vi "Master Sensor Update.vi"(11 "Input":T1={"GyroDevRef"={"DevStatus"={"status"=FALSE, "code"=0, "source"=""}, "Analog Channel"=enum."AI 1", "Offset"=0.0, "Gain (VoltsPerDegree/Second)"=0.0, "Gyro Type"=enum."Analog", "Handle"=0, "SPI Bus"=enum."Invalid", "Device Found"=FALSE, "Sample Rate"=1.0, "Calibrate On Open"=FALSE}, "Left Arm Limit DigitalInputDevRef"={"DevStatus"={"status"=FALSE, "code"=0, "source"=""}, "DIO Channel"=enum."DIO 1"}, "Right Arm Limit DigitalInputDevRef"={"DevStatus"={"status"=FALSE, "code"=0, "source"=""}, "DIO Channel"=enum."DIO 1"}, "Left Arm EncoderDevRef"={"DevStatus"={"status"=FALSE, "code"=0, "source"=""}, "EncoderIndex"=enum."Invalid", "CounterIndex"=enum."Invalid", "DistancePerCount"=1.0, "Decoding Type"=enum."4x"}, "Right Arm EncoderDevRef"={"DevStatus"={"status"=FALSE, "code"=0, "source"=""}, "EncoderIndex"=enum."Invalid", "CounterIndex"=enum."Invalid", "DistancePerCount"=1.0, "Decoding Type"=enum."4x"}, "Left Drive EncoderDevRef"={"DevStatus"={"status"=FALSE, "code"=0, "source"=""}, "EncoderIndex"=enum."Invalid", "CounterIndex"=enum."Invalid", "DistancePerCount"=1.0, "Decoding Type"=enum."4x"}, "Right Drive EncoderDevRef"={"DevStatus"={"status"=FALSE, "code"=0, "source"=""}, "EncoderIndex"=enum."Invalid", "CounterIndex"=enum."Invalid", "DistancePerCount"=1.0, "Decoding Type"=enum."4x"}, "BoB Photoeye DigitalInputDevRef"={"DevStatus"={"status"=FALSE, "code"=0, "source"=""}, "DIO Channel"=enum."DIO 1"}, "Range SonarMB1010AnalogDevRef"={"AIDeviceRef"={"DevStatus"={"status"=FALSE, "code"=0, "source"=""}, "Analog Channel"=enum."Invalid"}, "Scaling factor (V/in)"=0.0098, "Average Bits"=3}, "Shooter CounterDevRef"={"DevStatus"={"status"=FALSE, "code"=0, "source"=""}, "CntIndex"=enum."Invalid"}, "AccelerometerDevRef"={"DevStatus"={"status"=FALSE, "code"=0, "source"=""}, "Scaling"={"Gain (VoltsPerG)"=0.0, "Center Voltage"=0.0}, "Analog Channels"={"X-Axis"=enum."Invalid", "Y-Axis"=enum."Invalid", "Z-Axis"=enum."Invalid"}, "I2C Bus"=enum."Invalid", "SPI Bus"=enum."Invalid", "Accel Range"=0, "ADXL Axes"={"X-Axis"=FALSE, "Y-Axis"=FALSE, "Z-Axis"=FALSE}, "Handle"=0, "Device Address"=0, "Accel Type"=enum."Analog"}, "Left Hanging Erecter EncoderDevRef"={"DevStatus"={"status"=FALSE, "code"=0, "source"=""}, "EncoderIndex"=enum."Enc 0", "CounterIndex"=enum."Invalid", "DistancePerCount"=1.0, "Decoding Type"=enum."4x"}, "Right Hanging Erecter EncoderDevRef"={"DevStatus"={"status"=FALSE, "code"=0, "source"=""}, "EncoderIndex"=enum."Enc 1", "CounterIndex"=enum."Invalid", "DistancePerCount"=1.0, "Decoding Type"=enum."4x"}, "TestDigitalInputDevRef"={"DevStatus"={"status"=FALSE, "code"=0, "source"=""}, "DIO Channel"=enum."DIO 1"}} {"AccelerometerDevRef"."Device Address" format="%.0x"; "AccelerometerDevRef"."Accel Range" items=["+/- 2 g", "+/- 4 g", "+/- 8 g", "+/- 16 g"]; "Range SonarMB1010AnalogDevRef"."Average Bits" max=15; "GyroDevRef"."Sample Rate" min=0.25 max=100.0 step=0.25}) -> (3 "Output":T1={"GyroDevRef"={"DevStatus"={"status"=FALSE, "code"=0, "source"=""}, "Analog Channel"=enum."AI 1", "Offset"=0.0, "Gain (VoltsPerDegree/Second)"=0.0, "Gyro Type"=enum."Analog", "Handle"=0, "SPI Bus"=enum."Invalid", "Device Found"=FALSE, "Sample Rate"=1.0, "Calibrate On Open"=FALSE}, "Left Arm Limit DigitalInputDevRef"={"DevStatus"={"status"=FALSE, "code"=0, "source"=""}, "DIO Channel"=enum."DIO 1"}, "Right Arm Limit DigitalInputDevRef"={"DevStatus"={"status"=FALSE, "code"=0, "source"=""}, "DIO Channel"=enum."DIO 1"}, "Left Arm EncoderDevRef"={"DevStatus"={"status"=FALSE, "code"=0, "source"=""}, "EncoderIndex"=enum."Invalid", "CounterIndex"=enum."Invalid", "DistancePerCount"=1.0, "Decoding Type"=enum."4x"}, "Right Arm EncoderDevRef"={"DevStatus"={"status"=FALSE, "code"=0, "source"=""}, "EncoderIndex"=enum."Invalid", "CounterIndex"=enum."Invalid", "DistancePerCount"=1.0, "Decoding Type"=enum."4x"}, "Left Drive EncoderDevRef"={"DevStatus"={"status"=FALSE, "code"=0, "source"=""}, "EncoderIndex"=enum."Invalid", "CounterIndex"=enum."Invalid", "DistancePerCount"=1.0, "Decoding Type"=enum."4x"}, "Right Drive EncoderDevRef"={"DevStatus"={"status"=FALSE, "code"=0, "source"=""}, "EncoderIndex"=enum."Invalid", "CounterIndex"=enum."Invalid", "DistancePerCount"=1.0, "Decoding Type"=enum."4x"}, "BoB Photoeye DigitalInputDevRef"={"DevStatus"={"status"=FALSE, "code"=0, "source"=""}, "DIO Channel"=enum."DIO 1"}, "Range SonarMB1010AnalogDevRef"={"AIDeviceRef"={"DevStatus"={"status"=FALSE, "code"=0, "source"=""}, "Analog Channel"=enum."Invalid"}, "Scaling factor (V/in)"=0.0098, "Average Bits"=3}, "Shooter CounterDevRef"={"DevStatus"={"status"=FALSE, "code"=0, "source"=""}, "CntIndex"=enum."Invalid"}, "AccelerometerDevRef"={"DevStatus"={"status"=FALSE, "code"=0, "source"=""}, "Scaling"={"Gain (VoltsPerG)"=0.0, "Center Voltage"=0.0}, "Analog Channels"={"X-Axis"=enum."Invalid", "Y-Axis"=enum."Invalid", "Z-Axis"=enum."Invalid"}, "I2C Bus"=enum."Invalid", "SPI Bus"=enum."Invalid", "Accel Range"=0, "ADXL Axes"={"X-Axis"=FALSE, "Y-Axis"=FALSE, "Z-Axis"=FALSE}, "Handle"=0, "Device Address"=0, "Accel Type"=enum."Analog"}, "Left Hanging Erecter EncoderDevRef"={"DevStatus"={"status"=FALSE, "code"=0, "source"=""}, "EncoderIndex"=enum."Enc 0", "CounterIndex"=enum."Invalid", "DistancePerCount"=1.0, "Decoding Type"=enum."4x"}, "Right Hanging Erecter EncoderDevRef"={"DevStatus"={"status"=FALSE, "code"=0, "source"=""}, "EncoderIndex"=enum."Enc 1", "CounterIndex"=enum."Invalid", "DistancePerCount"=1.0, "Decoding Type"=enum."4x"}, "TestDigitalInputDevRef"={"DevStatus"={"status"=FALSE, "code"=0, "source"=""}, "DIO Channel"=enum."DIO 1"}} {"AccelerometerDevRef"."Device Address" format="%.0x"; "AccelerometerDevRef"."Accel Range" items=["+/- 2 g", "+/- 4 g", "+/- 8 g", "+/- 16 g"]; "Range SonarMB1010AnalogDevRef"."Average Bits" max=15; "GyroDevRef"."Sample Rate" min=0.25 max=100.0 step=0.25})   [LabVIEW 2015]
uses:
  Sensors.ctl
  <vilib>/Rock Robotics/WPI/Gyro/WPI_GyroDevRef.ctl
  <vilib>/Rock Robotics/SystemInterfaces/AI/FPGA_AIChannel.ctl
  <vilib>/Rock Robotics/SystemInterfaces/spilib/spi_bus.ctl
  <vilib>/Rock Robotics/WPI/DigitalInput/WPI_DigitalInputDevRef.ctl
  <vilib>/Rock Robotics/SystemInterfaces/DIO/FPGA_DIOChannel.ctl
  <vilib>/Rock Robotics/WPI/Encoder/WPI_EncoderDevRef.ctl
  <vilib>/Rock Robotics/SystemInterfaces/Encoder/FPGA_EncoderIdx.ctl
  <vilib>/Rock Robotics/SystemInterfaces/Counter/FPGA_CounterCtrSystemIndex.ctl
  <vilib>/Rock Robotics/WPI/Encoder/WPI_EncoderType.ctl
  <vilib>/Rock Robotics/WPI/Ultrasonic/WPI_SonarMB1010AnalogDeviceRef.ctl
  <vilib>/Rock Robotics/WPI/AnalogChannel/WPI_AnalogChannelDevRef.ctl
  <vilib>/Rock Robotics/WPI/Counter/WPI_CounterDevRef.ctl
  <vilib>/Rock Robotics/WPI/Accelerometer/WPI_AccelerometerDevRef.ctl
  <vilib>/Rock Robotics/WPI/Accelerometer/WPI_AccelerometerScaling.ctl
  <vilib>/Rock Robotics/WPI/Accelerometer/WPI_AccelerometerAnalogChannels.ctl
  <vilib>/Rock Robotics/SystemInterfaces/i2clib/i2c_bus.ctl
  <vilib>/Rock Robotics/WPI/Accelerometer/ADXL345 Range.ctl
  <vilib>/Rock Robotics/WPI/Accelerometer/WPI_AccelerometerADXL345 Axes.ctl
  <vilib>/Rock Robotics/Network Tables/NT Write Number.vi
  <vilib>/Rock Robotics/Network Tables/NT Read Numeric Array.vi
  <vilib>/Rock Robotics/Network Tables/NT Write Boolean.vi
  <vilib>/Rock Robotics/Network Tables/NT Read Boolean.vi
  Robot Values.vi
  <vilib>/Rock Robotics/WPI/Ultrasonic/WPI_SonarMB1010AnalogGetRange.vi
panel:
  in  "Gyro Multiplier":dbl=1.125 format="%#_13g"
  # "ADXL"
  # "Analog"
  # "Analog"
  # "XRS"
  # "ADXL"
  # "Analog"
  # "Analog"
  # "XRS"
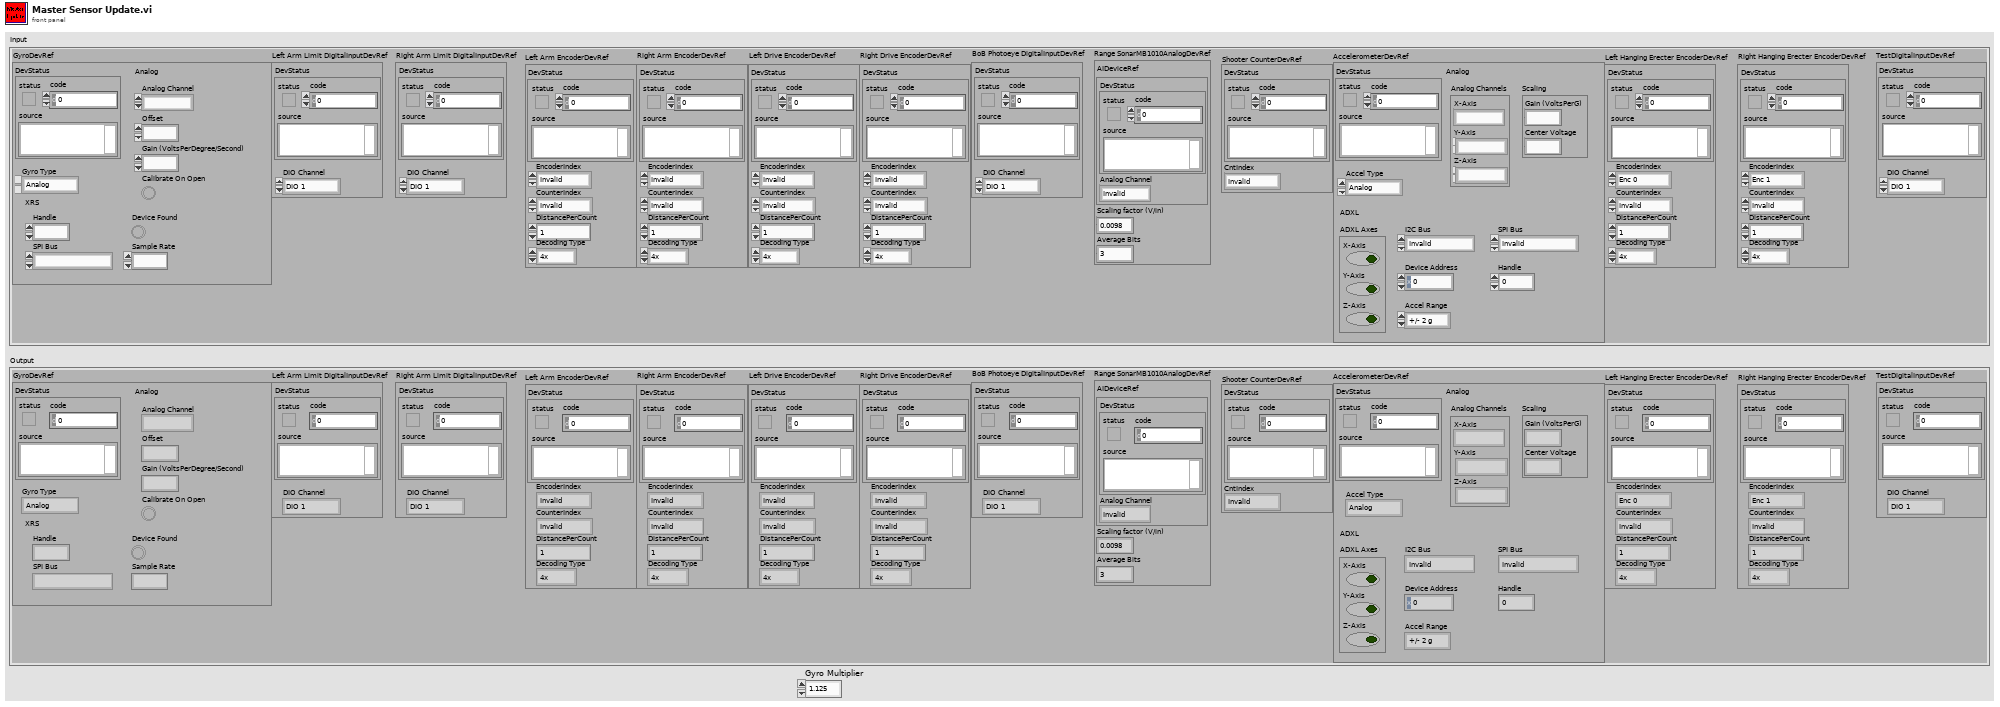
[diagram p1: front panel]
types:
  T1 = typedef "Sensors.ctl" = cluster{"GyroDevRef":T2, "Left Arm Limit DigitalInputDevRef":T5, "Right Arm Limit DigitalInputDevRef":T5, "Left Arm EncoderDevRef":T7, "Right Arm EncoderDevRef":T7, "Left Drive EncoderDevRef":T7, "Right Drive EncoderDevRef":T7, "BoB Photoeye DigitalInputDevRef":T5, "Range SonarMB1010AnalogDevRef":T11, "Shooter CounterDevRef":T13, "AccelerometerDevRef":T14, "Left Hanging Erecter EncoderDevRef":T7, "Right Hanging Erecter EncoderDevRef":T7, "TestDigitalInputDevRef":T5}
  T2 = typedef "WPI_GyroDevRef.ctl" = cluster{"DevStatus":errorcluster, "Analog Channel":T3, "Offset":dbl, "Gain (VoltsPerDegree/Second)":dbl, "Gyro Type":enum16{"Analog", "XRS450"}, "Handle":i32, "SPI Bus":T4, "Device Found":bool, "Sample Rate":dbl, "Calibrate On Open":bool}
  T3 = typedef "FPGA_AIChannel.ctl" = enum8{"AI 0", "AI 1", "AI 2", "AI 3", "AI MXP 0", "AI MXP 1", "AI MXP 2", "AI MXP 3", "Invalid"}
  T4 = typedef "spi_bus.ctl" = enum16{"SPI On-Board, CS0", "SPI On-Board, CS1", "SPI On-Board, CS2", "SPI On-Board, CS3", "SPI MXP", "Invalid"}
  T5 = typedef "WPI_DigitalInputDevRef.ctl" = cluster{"DevStatus":errorcluster, "DIO Channel":T6}
  T6 = typedef "FPGA_DIOChannel.ctl" = enum8{"DIO 0", "DIO 1", "DIO 2", "DIO 3", "DIO 4", "DIO 5", "DIO 6", "DIO 7", "DIO 8", "DIO 9", "DIO MXP 0", "DIO MXP 1", "DIO MXP 2", "DIO MXP 3", "DIO MXP 4", "DIO MXP 5", "DIO MXP 6", "DIO MXP 7", "DIO MXP 8", "DIO MXP 9", "DIO MXP 10", "DIO MXP 11", "DIO MXP 12", "DIO MXP 13", "DIO MXP 14", "DIO MXP 15", "Invalid"}
  T7 = typedef "WPI_EncoderDevRef.ctl" = cluster{"DevStatus":errorcluster, "EncoderIndex":T8, "CounterIndex":T9, "DistancePerCount":dbl, "Decoding Type":T10}
  T8 = typedef "FPGA_EncoderIdx.ctl" = enum8{"Enc 0", "Enc 1", "Enc 2", "Enc 3", "Enc 4", "Enc 5", "Enc 6", "Enc 7", "Invalid"}
  T9 = typedef "FPGA_CounterCtrSystemIndex.ctl" = enum8{"Ctr 0", "Ctr 1", "Ctr 2", "Ctr 3", "Ctr 4", "Ctr 5", "Ctr 6", "Ctr 7", "Invalid"}
  T10 = typedef "WPI_EncoderType.ctl" = enum16{"1x", "2x", "4x"}
  T11 = typedef "WPI_SonarMB1010AnalogDeviceRef.ctl" = cluster{"AIDeviceRef":T12, "Scaling factor (V/in)":dbl, "Average Bits":u8}
  T12 = typedef "WPI_AnalogChannelDevRef.ctl" = cluster{"DevStatus":errorcluster, "Analog Channel":T3}
  T13 = typedef "WPI_CounterDevRef.ctl" = cluster{"DevStatus":errorcluster, "CntIndex":T9}
  T14 = typedef "WPI_AccelerometerDevRef.ctl" = cluster{"DevStatus":errorcluster, "Scaling":T15, "Analog Channels":T16, "I2C Bus":T17, "SPI Bus":T4, "Accel Range":T18, "ADXL Axes":T19, "Handle":i32, "Device Address":u8, "Accel Type":enum16{"Analog", "ADXL345 I2C", "ADXL345 SPI", "Internal", "ADXL362 SPI"}}
  T15 = typedef "WPI_AccelerometerScaling.ctl" = cluster{"Gain (VoltsPerG)":dbl, "Center Voltage":dbl}
  T16 = typedef "WPI_AccelerometerAnalogChannels.ctl" = cluster{"X-Axis":T3, "Y-Axis":T3, "Z-Axis":T3}
  T17 = typedef "i2c_bus.ctl" = enum16{"I2C On-Board", "I2C MXP", "Invalid"}
  T18 = typedef "ADXL345 Range.ctl" = u8
  T19 = typedef "WPI_AccelerometerADXL345 Axes.ctl" = cluster{"X-Axis":bool, "Y-Axis":bool, "Z-Axis":bool}
  T20 = typedef "Robot Values.ctl" = cluster{"Drive Motors":cluster{"Left Motor Value":dbl, "Right Motor Value":dbl, "Left Motor Encoder":dbl, "Right Motor Encoder":dbl, "High/Low Gear":bool}, "Sensors":cluster{"Gyro Angle":dbl, "Photoeye":bool, "Ultrasonic Range":dbl, "Shooter Speed Encoder":dbl, "Accelerometer Value":dbl, "Flashlight":bool, "Target Distance":dbl, "Target X Value":dbl, "Reset Gyro?":bool}, "Arms":cluster{"Desired Arm Position":dbl, "Left Arm Encoder":dbl, "Right Arm Encoder":dbl, "Left Arm Lower Limit":bool, "Right Arm Lower Limit":bool, "Initialize Arm Position?":bool}, "Acquisition and Scoring":cluster{"Acquiring?":bool, "Current Speed":dbl, "Setpoint Speed":dbl, "Prep Wheels":bool, "Shoot":bool, "Low Eject":bool, "Reverse Shooter Wheel":bool}, "Hanging":cluster{"Pivot Arms":dbl, "PTO":bool, "Left Pivot Encoder":dbl, "Right Pivot Encoder":dbl, "Hanging Pin":bool}}
  T21 = cluster{"X-Axis":dbl, "Y-Axis":dbl, "Z-Axis":dbl}
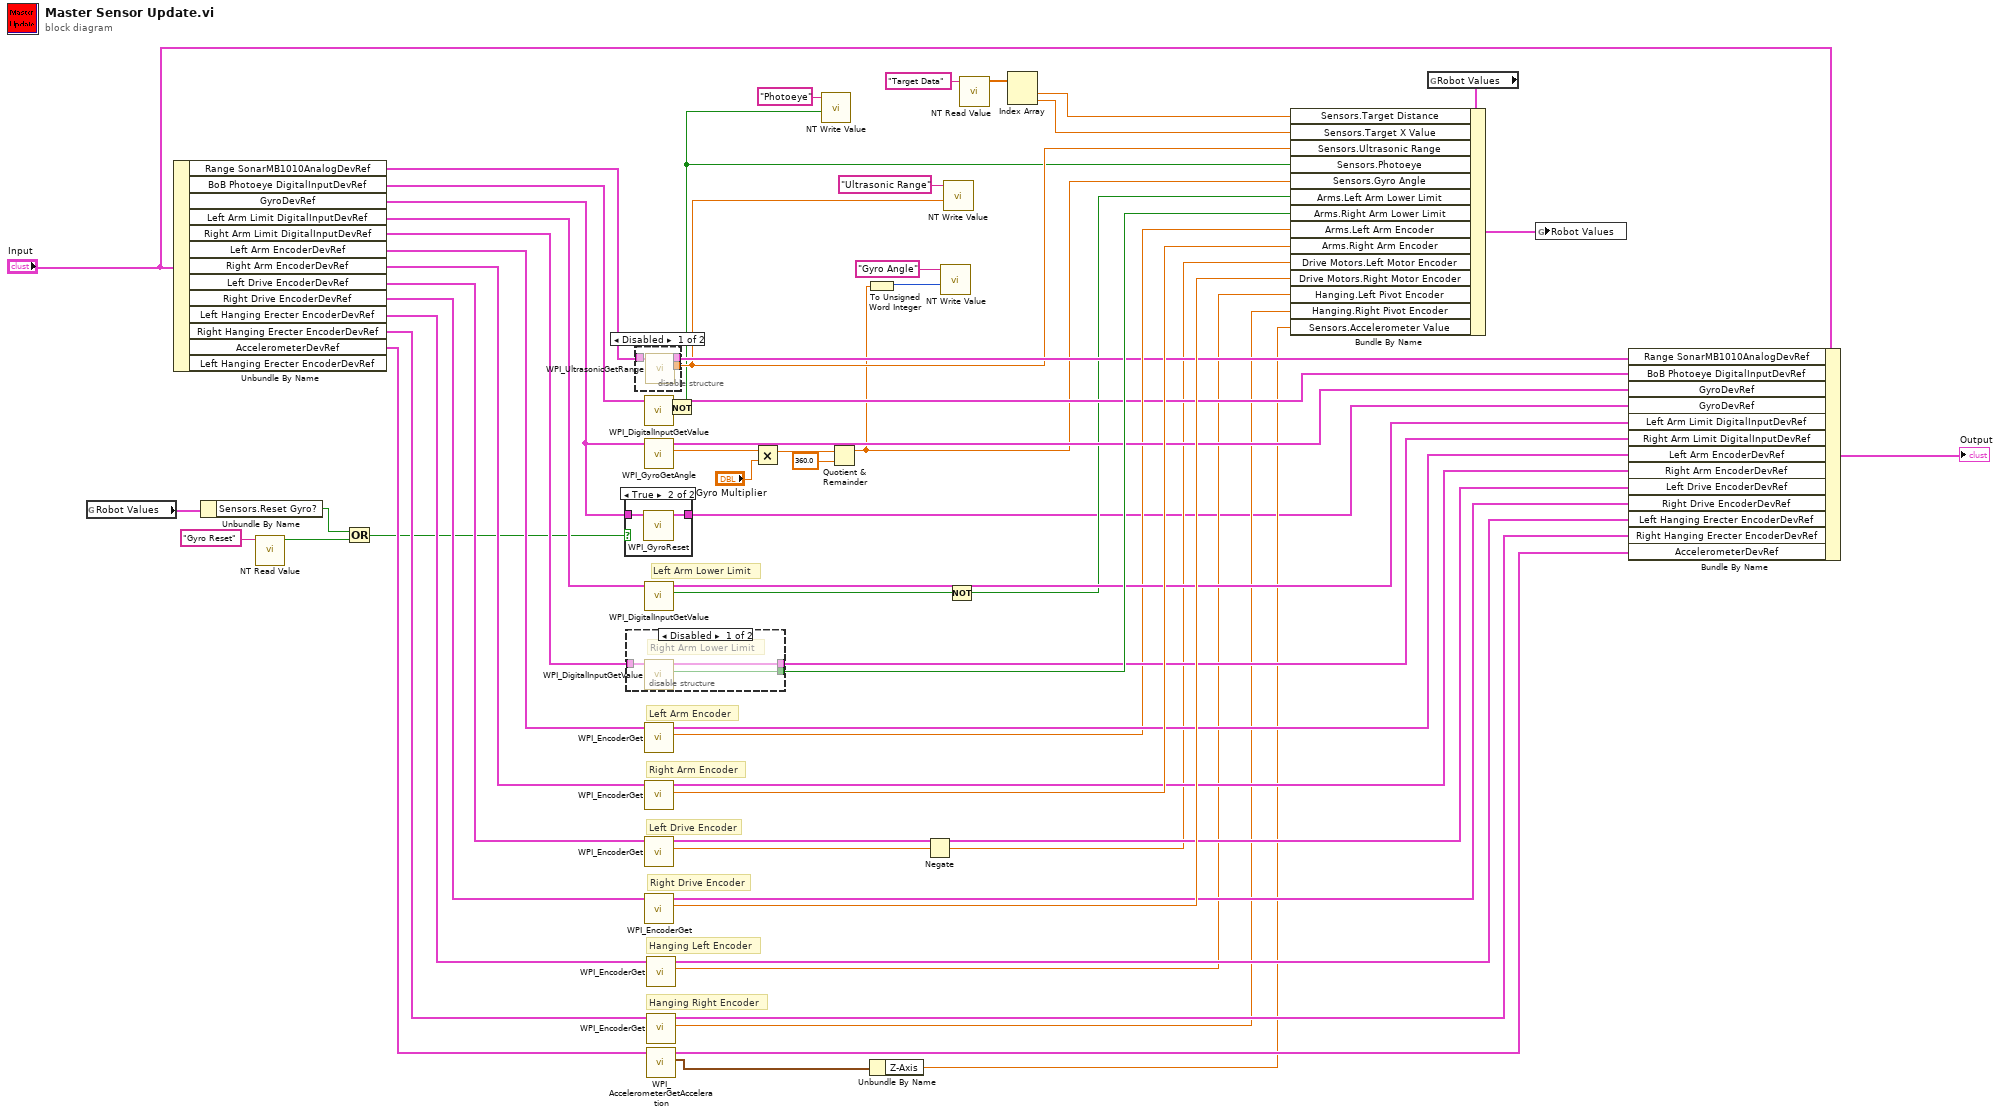
[diagram p0: block diagram]
diagram:
  # "Hanging Right Encoder"
  # "Hanging Left Encoder"
  # "Right Drive Encoder"
  # "Left Drive Encoder"
  # "Right Arm Encoder"
  # "Left Arm Encoder"
  # "Left Arm Lower Limit"
  n1 = global read "Robot Values.vi" "Robot Values"() -> (w11:T20)
  n2 = Unbundle By Name("Input") -> ("Range SonarMB1010AnalogDevRef"=w37:T11, "BoB Photoeye DigitalInputDevRef"=w39:T5, "GyroDevRef"=w13:T2, "Left Arm Limit DigitalInputDevRef"=w57:T5, "Right Arm Limit DigitalInputDevRef"=w56:T5, "Left Arm EncoderDevRef"=w55:T7, "Right Arm EncoderDevRef"=w54:T7, "Left Drive EncoderDevRef"=w53:T7, "Right Drive EncoderDevRef"=w52:T7, "Left Hanging Erecter EncoderDevRef"=w51:T7, "Right Hanging Erecter EncoderDevRef"=w31:T7, "AccelerometerDevRef"=w28:T14)  [unwired: 1 out]
  n3 = Unbundle By Name(w11) -> ("Sensors.Reset Gyro?"=w10:bool)
  n4 = call-poly <vilib>:"NT Read Value.vi"("Name"="Gyro Reset") -> ("Boolean"=w4:bool)  [unwired: 9 in, 1 out]
  n5 = Or(x=w10, y=w4) -> (x .or. y?=w5:bool)
  n6 = case shown="True" w5 {
    tunnel: [w63 w65] -> w12
    tunnel: w13 -> [w63 w64]
    frame False {
    }
    frame True {
      n7 = call <vilib>:"WPI_GyroReset.vi"("GyroDevRef"=w64) -> ("GyroDevRef"=w65:T2)  [unwired: 9 in, 1 out]
    }
  }
  n8 = disable-structure shown="Disabled" {
    disable-tunnel: [w68 _] -> w58
    disable-tunnel: w56 -> [w67 _]
    disable-tunnel: [w66 _] -> w45
    frame Disabled {
      # "Right Arm Lower Limit"
      n9 = call <vilib>:"WPI_DigitalInputGetValue.vi"("DigitalInputDevRef"=w67) -> ("Value"=w68:bool, "DigitalInputDevRef"=w66:T5)  [unwired: 8 in, 1 out]
    }
    frame Enabled {
    }
  }
  n10 = disable-structure shown="Disabled" {
    disable-tunnel: w37 -> [w71 _]
    disable-tunnel: [w70 _] -> w36
    disable-tunnel: [w69 _] -> w35
    frame Disabled {
      n11 = call-poly <vilib>:"WPI_UltrasonicGetRange.vi"("SonarMB1010AnalogDevRef"=w71) -> ("Distance"=w69:dbl, "SonarMB1010AnalogDevRef"=w70:T11)  [unwired: 8 in, 1 out]
    }
    frame Enabled {
    }
  }
  n12 = call <vilib>:"WPI_DigitalInputGetValue.vi"("DigitalInputDevRef"=w39) -> ("Value"=w17:bool, "DigitalInputDevRef"=w38:T5)  [unwired: 8 in, 1 out]
  n13 = call <vilib>:"WPI_GyroGetAngle.vi"("GyroDevRef"=w13) -> ("Angle"=w9:dbl, "GyroDevRef"=w47:T2)  [unwired: 6 in, 3 out]
  n14 = call <vilib>:"WPI_DigitalInputGetValue.vi"("DigitalInputDevRef"=w57) -> ("Value"=w59:bool, "DigitalInputDevRef"=w46:T5)  [unwired: 8 in, 1 out]
  n15 = call <vilib>:"WPI_EncoderGet.vi"("EncoderDevRef"=w55) -> ("Distance"=w40:dbl, "EncoderDevRef"=w44:T7)  [unwired: 5 in, 4 out]
  n16 = call <vilib>:"WPI_EncoderGet.vi"("EncoderDevRef"=w54) -> ("Distance"=w50:dbl, "EncoderDevRef"=w43:T7)  [unwired: 5 in, 4 out]
  n17 = call <vilib>:"WPI_EncoderGet.vi"("EncoderDevRef"=w53) -> ("Distance"=w49:dbl, "EncoderDevRef"=w42:T7)  [unwired: 5 in, 4 out]
  n18 = call <vilib>:"WPI_EncoderGet.vi"("EncoderDevRef"=w52) -> ("Distance"=w48:dbl, "EncoderDevRef"=w41:T7)  [unwired: 5 in, 4 out]
  n19 = call <vilib>:"WPI_EncoderGet.vi"("EncoderDevRef"=w51) -> ("Distance"=w24:dbl, "EncoderDevRef"=w30:T7)  [unwired: 5 in, 4 out]
  n20 = call <vilib>:"WPI_EncoderGet.vi"("EncoderDevRef"=w31) -> ("Distance"=w23:dbl, "EncoderDevRef"=w29:T7)  [unwired: 5 in, 4 out]
  n21 = call <vilib>:"WPI_AccelerometerGetAcceleration.vi"("AccelerometerDevRef"=w28) -> ("Accelerations"=w26:T21, "AccelerometerDevRef"=w27:T14)  [unwired: 8 in, 1 out]
  n22 = Not(x=w17) -> (.not. x?=w7:bool)
  n23 = Multiply(x=w9, y="Gyro Multiplier") -> (x*y=w2:dbl)
  n24 = call-poly <vilib>:"NT Write Value.vi"("Boolean"=w7, "Name"="Photoeye") -> ()  [unwired: 9 in, 1 out]
  n25 = Quotient & Remainder(x=w2, y=360.0) -> (x-y*floor(x/y)=w8:dbl)  [unwired: 1 out]
  n26 = To Unsigned Word Integer(number=w8) -> (unsigned 16bit integer=w6:u16)
  n27 = Unbundle By Name(w26) -> ("Z-Axis"=w25:dbl)
  n28 = Negate(x=w49) -> (-x=w14:dbl)
  n29 = call-poly <vilib>:"NT Write Value.vi"("Numeric"=w6, "Name"="Gyro Angle") -> ()  [unwired: 9 in, 1 out]
  n30 = call-poly <vilib>:"NT Write Value.vi"("Numeric"=w35, "Name"="Ultrasonic Range") -> ()  [unwired: 9 in, 1 out]
  n31 = Not(x=w59) -> (.not. x?=w15:bool)
  n32 = call-poly <vilib>:"NT Read Value.vi"("Name"="Target Data") -> ("Numeric Array"=w21:dbl[])  [unwired: 9 in, 1 out]
  n33 = Index Array(array=w21) -> (element #1=w20:dbl, element #2=w19:dbl)  [unwired: 2 in]
  n34 = global read "Robot Values.vi" "Robot Values"() -> (w62:T20)
  n35 = Bundle By Name(cluster=w62, "Sensors.Target Distance"=w20, "Sensors.Target X Value"=w19, "Sensors.Ultrasonic Range"=w35, "Sensors.Photoeye"=w7, "Sensors.Gyro Angle"=w8, "Arms.Left Arm Lower Limit"=w15, "Arms.Right Arm Lower Limit"=w58, "Arms.Left Arm Encoder"=w40, "Arms.Right Arm Encoder"=w50, "Drive Motors.Left Motor Encoder"=w14, "Drive Motors.Right Motor Encoder"=w48, "Hanging.Left Pivot Encoder"=w24, "Hanging.Right Pivot Encoder"=w23, "Sensors.Accelerometer Value"=w25) -> (w61:T20)
  n36 = global write "Robot Values.vi" "Robot Values"(w61) -> ()
  n37 = Bundle By Name(cluster="Input", "Range SonarMB1010AnalogDevRef"=w36, "BoB Photoeye DigitalInputDevRef"=w38, "GyroDevRef"=w47, "GyroDevRef"=w12, "Left Arm Limit DigitalInputDevRef"=w46, "Right Arm Limit DigitalInputDevRef"=w45, "Left Arm EncoderDevRef"=w44, "Right Arm EncoderDevRef"=w43, "Left Drive EncoderDevRef"=w42, "Right Drive EncoderDevRef"=w41, "Left Hanging Erecter EncoderDevRef"=w30, "Right Hanging Erecter EncoderDevRef"=w29, "AccelerometerDevRef"=w27) -> (→"Output":T1)
